vi "Agilent PWM Set Zeroing Type.vi"(7 "Agilent PWM":T1, 8 "error in (no error)":errorcluster, 10 "Frequency (MHz)":enum16{"Internal", "External"}(ring), 11 "VISA Resource Name":refnum<visa-resource-name>) -> (0 "error out":errorcluster, 3 "dup VISA Resource Name":refnum<visa-resource-name>)   [LabVIEW 2011]
doc: "This VI for the HP 8753 is used to read the sweep type.\n\n0 LINEAR FREQ\n1 LOG FREQ\n2 LIST FREQ\n3 CW TIME\n4 POWER SWEEP"
uses:
  TypeDefs/Agilent PWM Instrument Info.ctl
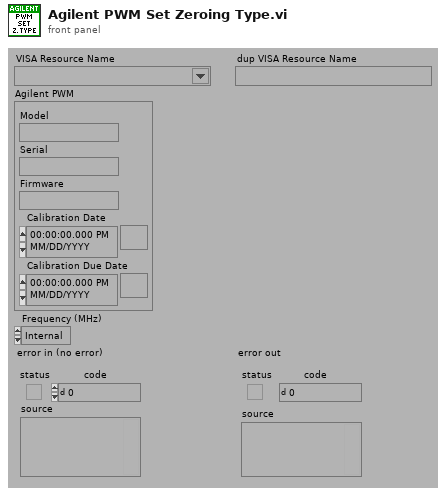
[diagram p1: front panel]
types:
  T1 = typedef "Agilent PWM Instrument Info.ctl" = cluster{"Model":string, "Serial":string, "Firmware":string, "Calibration Date":timestamp, "Calibration Due Date":timestamp}
  T2 = typedef "Agilent PWM Model.ctl" = enum16{"Not Supported", "E4418X", "E4419X", "U2000X"}
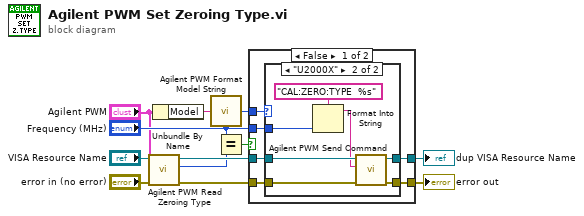
[diagram p0: block diagram]
diagram:
  n1 = call "Agilent PWM Read Zeroing Type.vi"("Agilent PWM"="Agilent PWM", "error in (no error)"="error in (no error)", "VISA Resource Name"="VISA Resource Name") -> ("error out"=w9:errorcluster, "Frequency (MHz)"=w5:enum16{"Internal", "External"}, "dup VISA Resource Name"=w8:refnum<visa-resource-name>)  [unwired: 6 in]
  n2 = Unbundle By Name("Agilent PWM") -> ("Model"=w3:string)
  n3 = call "Agilent PWM Format Model String.vi"("Model"=w3) -> ("Model"=w1:T2)
  n4 = Equal?(x="Frequency (MHz)", y=w5) -> (x = y?=w10:bool)
  n5 = case shown="False" w10 {
    tunnel: [w18 w29] -> w7
    tunnel: [w17 w28] -> w6
    tunnel: w8 -> [w16 w29]
    tunnel: w9 -> [w15 w28]
    tunnel: "Frequency (MHz)" -> [w14 _]
    tunnel: w1 -> [w13 _]
    frame False {
      n6 = case shown="\"U2000X\"" w13 {
        tunnel: [w20 w27] -> w18
        tunnel: [w19 w26] -> w17
        tunnel: w16 -> [w20 w25]
        tunnel: w15 -> [w19 w24]
        tunnel: w14 -> [_ w21]
        frame "Not Supported", "E4418X", Default {
        }
        frame "U2000X" {
          n7 = Format Into String(format string="CAL:ZERO:TYPE  %s" ("write buffer"), w21) -> (resulting string=w22:string)  [unwired: 2 in, 1 out]
          n8 = call "Agilent PWM Send Command.vi"("error in (no error)"=w24, "Command"=w22, "VISA Resource Name"=w25) -> ("error out"=w26:errorcluster, "dup VISA Resource Name"=w27:refnum<visa-resource-name>)  [unwired: 2 in, 5 out]
        }
      }
    }
    frame True {
    }
  }
  "dup VISA Resource Name" <- w7
  "error out" <- w6
